vi "crc16 x8005.vi"(4 "message":string) -> (1 "CRC16":string)   [LabVIEW 2017]
doc: "This VI computes a CRC16 checksum from <B>message</B>.\nFor compatibility with the MODbus protocol the hi and low bytes of the CRC are swapped.\nThis crc16 uses the polynom 8005, i.e. x^16+x^15+x^2+1"
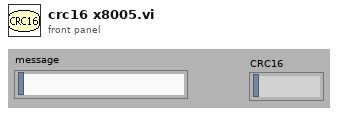
[diagram p1: front panel]
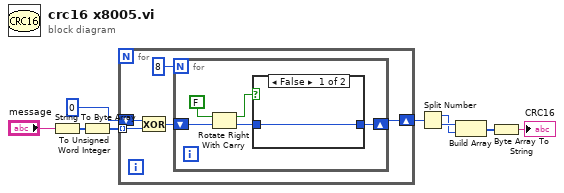
[diagram p0: block diagram]
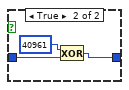
[diagram p2: hidden frame]
diagram:
  n1 = String To Byte Array(string="message") -> (unsigned byte array=w7:u8[])
  n2 = To Unsigned Word Integer(number=w7) -> (unsigned 16bit integer=w5:u16[])
  n3 = for {
    shift-right: [w11] -> w8
    shift-left: u16 0 -> [w12]
    tunnel: w5 -> [w10] mode=indexing
    n4 = Exclusive Or(1:w10, 2:w12) -> (0:w13:u16)
    n5 = for {
      N: 8 -> [_]
      shift-right: [w18] -> w11
      shift-left: w13 -> [w17]
      n6 = Rotate Right With Carry(2:w17, 3:FALSE ("Übertrag")) -> (0:w19:u16, 1:w16:bool)
      n7 = case shown="False" w16 {
        tunnel: w19 -> [w20 w22]
        tunnel: [w20 w21] -> w18
        frame False {
        }
        frame True {
          n8 = Exclusive Or(1:w22, 2:u16 40961) -> (0:w21:u16)
        }
      }
    }
  }
  n9 = Split Number(x=w8) -> (hi(x)=w3:u8, lo(x)=w4:u8)
  n10 = Build Array(w4, w3) -> (w2:u8[])
  n11 = Byte Array To String(unsigned byte array=w2) -> (string=→"CRC16":string)
